vi "Prepare User Input.vi"(11 "cluster":T1) -> (0 "error out":errorcluster)   [LabVIEW 2025]
doc: "Prepare the user input field (next to the \"E\" key). Clears it out and makes it the key focus."
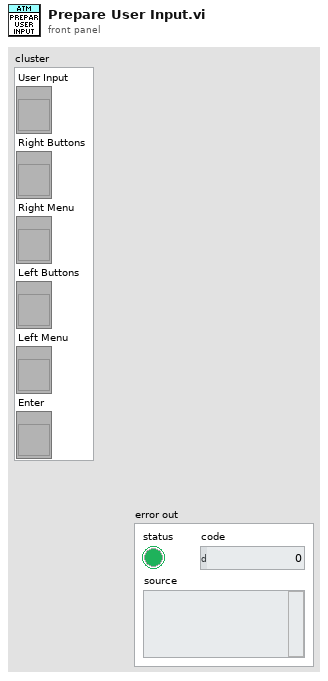
[diagram p1: front panel]
types:
  T1 = cluster{"User Input":refnum<vi>, "Right Buttons":refnum<vi>, "Right Menu":refnum<vi>, "Left Buttons":refnum<vi>, "Left Menu":refnum<vi>, "Enter":refnum<vi>}
  T2 = enum8{"Enabled", "Disabled", "Disabled and Grayed Out"}
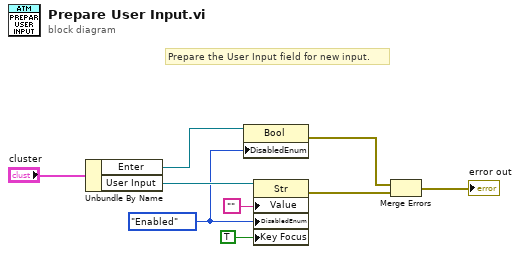
[diagram p0: block diagram]
diagram:
  w7 = T2."Enabled" ("Disabled")
  # "Prepare the User Input field for new input."
  n1 = Unbundle By Name("cluster") -> ("Enter"=w9:refnum<vi>, "User Input"=w8:refnum<vi>)
  n2 = property on="Property Node" class="Bool"(reference=w9, "DisabledEnum"=w7) -> (error out=w3:errorcluster)  [unwired: 1 in, 1 out]
  n3 = property on="Property Node" class="Str"(reference=w8, "Value"="" ("Empty String Constant"), "DisabledEnum"=w7, "Key Focus"=TRUE) -> (error out=w2:errorcluster)  [unwired: 1 in, 1 out]
  n4 = Merge Errors(w3, w2) -> (→"error out":errorcluster)
